vi "Connection Monitor - Loop.vi"(8 "error in (no error)":errorcluster, 11 "RemoteControl.STM in":refnum<class "RemoteControl.STM.lvclass">) -> (0 "error out":errorcluster, 3 "RemoteControl.STM out":refnum<class "RemoteControl.STM.lvclass">)   [LabVIEW 2016, in "RemoteControl.STM.lvclass"]
uses:
  RemoteControl.STM.lvclass
  <vilib>/NI/STM/Connection Manager/TCP/TCP Connection Method.ctl
  <vilib>/NI/STM/TCP/Write Meta Data (TCP Ref).vi
  <vilib>/NI/STM/TCP/Write Meta Data (TCP Clst).vi
  <userlib>/_OpenG.lib/error/error.llb/Filter Error Codes (Array)__ogtk.vi
  <vilib>/NI/STM/NI STM.lvlib
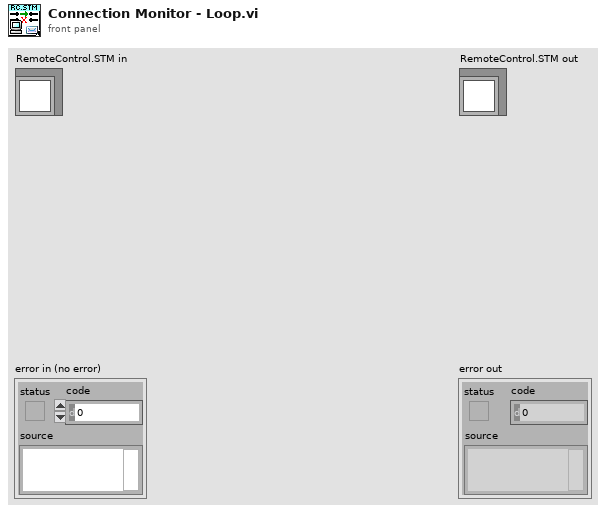
[diagram p1: front panel]
types:
  T1 = typedef "NI STM.lvlib/TCP Connection Method.ctl" = enum16{"Initialize", "Add Connection", "Set Properties", "Get Connection(s)", "Remove Connection", "Remove All Connections", "Get Connection Count"}
  T2 = typedef "NI STM.lvlib/TCP Connection Info.ctl" = cluster{"connection ID":refnum<k5>, "meta data":T3[]}
  T3 = typedef "NI STM.lvlib/MetaDataElement.ctl" = string
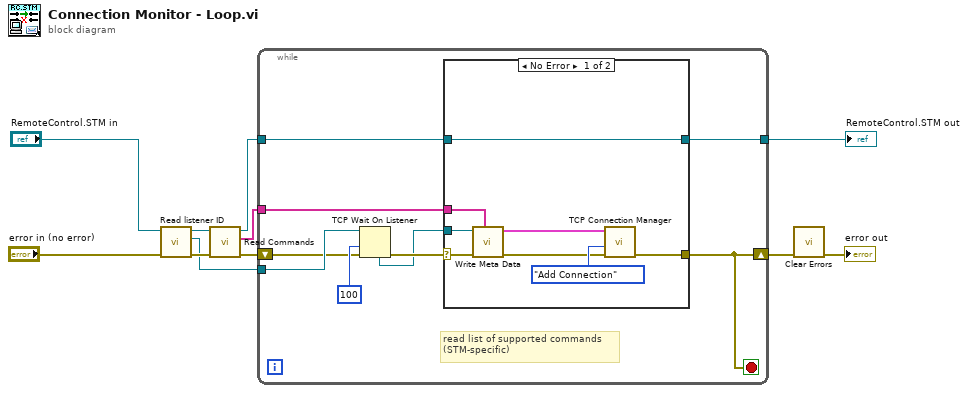
[diagram p0: block diagram]
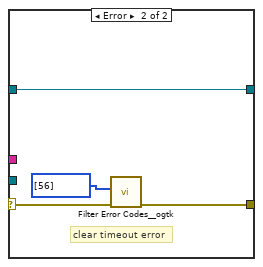
[diagram p2: hidden frame]
diagram:
  n1 = call-dynamic "Read listener ID.vi"("error in (no error)"="error in (no error)", "RemoteControl.STM in"="RemoteControl.STM in") -> ("error out"=w8:errorcluster, "listener ID"=w6:refnum<k5>, "RemoteControl.STM out"=w4:refnum<class "RemoteControl.STM.lvclass">)  [unwired: 7 in]
  n2 = call-dynamic "Read Commands.vi"("error in (no error)"=w8, "RemoteControl in"=w4) -> ("error out"=w9:errorcluster, "Commands"=w5:string[], "RemoteControl out"=w2:refnum<class "RemoteControl.STM.lvclass">)  [unwired: 7 in]
  n3 = while {
    shift-right: [w17] -> w11
    shift-left: w9 -> [w13]
    tunnel: w6 -> [w16]
    tunnel: w5 -> [w15]
    tunnel: w2 -> [w14]
    tunnel: [w18] -> w10
    stop <- w17 stop-if-true
    # "read list of supported commands\n(STM-specific)"
    n4 = TCP Wait On Listener(8:w13, 9:100 ("timeout ms (wait forever: -1)"), 11:w16) -> (0:w20:errorcluster, 4:w12:refnum<k5>)  [unwired: 1 in, 3 out]
    n5 = case shown="No Error" w20 {
      selector: w20 -> [w21 w31]
      tunnel: w12 -> [w28 _]
      tunnel: [w25 w30] -> w17
      tunnel: [w22 w29] -> w18
      tunnel: w14 -> [w22 w29]
      tunnel: w15 -> [w23 _]
      frame No Error {
        n6 = call-poly <vilib>:"Write Meta Data.vi"("meta data"=w23, "error in"=w21, "connection ID"=w28) -> ("error out"=w26:errorcluster, "connection info out"=w24:T2)  [unwired: 7 in]
        n7 = call <vilib>:"TCP Connection Manager.vi"("error in"=w26, "method"=TCP_Connection_Method."Add Connection", "connection in"=w24) -> ("error out"=w25:errorcluster)  [unwired: 3 in, 5 out]
      }
      frame Error {
        # "clear timeout error"
        n8 = call-poly <userlib>:"Filter Error Codes__ogtk.vi"("Error In"=w31, "Error Codes to Filter"=i32[] [56]) -> ("Error Out"=w30:errorcluster)  [unwired: 7 in, 2 out]
      }
    }
  }
  "RemoteControl.STM out" <- w10
  n9 = call <vilib>:"Clear Errors.vi"("error in (no error)"=w11) -> ("error out"=→"error out":errorcluster)  [unwired: 5 in, 1 out]
